vi "VannaSelection.vi"(2 "Vanna Motor":i16) -> (0 "Vanna Teleop Command":T1)   [LabVIEW 2019]
uses:
  Vanna Mode Type Def.ctl
  Vanna Command Type Def.ctl
panel:
  # "Operator Right joystick X: Vanna Manual. must have deadband.\nOperator Left Joystick Y: UP = Rotation control; DOWN = position control"
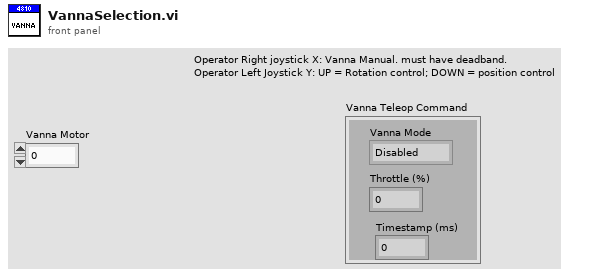
[diagram p1: front panel]
types:
  T1 = typedef "Vanna Command Type Def.ctl" = cluster{"Vanna Mode":T2, "Throttle (%)":dbl, "Timestamp (ms)":dbl}
  T2 = typedef "Vanna Mode Type Def.ctl" = enum16{"Disabled", "Raw Throttle", "Rotation Control", "Position Control"}
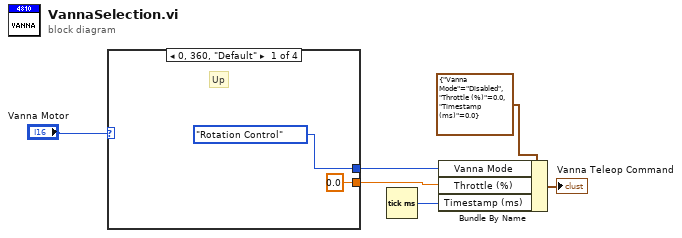
[diagram p0: block diagram]
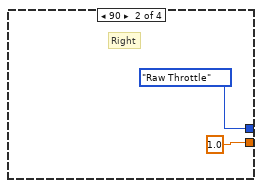
[diagram p2: hidden frame]
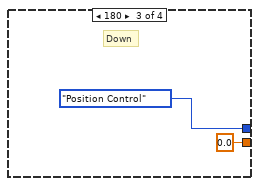
[diagram p3: hidden frame]
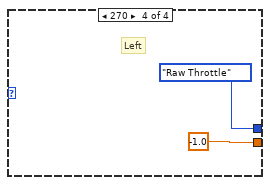
[diagram p4: hidden frame]
diagram:
  n1 = case shown="0, 360, \"Default\"" "Vanna Motor" {
    tunnel: [Vanna_Mode_Type_Def."Rotation Control" ("Vanna Mode") Vanna_Mode_Type_Def."Raw Throttle" ("Vanna Mode") Vanna_Mode_Type_Def."Position Control" ("Vanna Mode") Vanna_Mode_Type_Def."Raw Throttle" ("Vanna Mode")] -> w2
    tunnel: [0.0 ("Throttle (%)") 1.0 ("Throttle (%)") 0.0 ("Throttle (%)") -1.0 ("Throttle (%)")] -> w1
    frame 0, 360, 0 {
      # "Up"
    }
    frame 90 {
      # "Right"
    }
    frame 180 {
      # "Down"
    }
    frame 270 {
      # "Left"
    }
  }
  n2 = Tick Count (ms)() -> (millisecond timer value=w5:u32)
  n3 = Bundle By Name(cluster=T1 {"Vanna Mode"=enum."Disabled", "Throttle (%)"=0.0, "Timestamp (ms)"=0.0} ("Vanna Command"), "Vanna Mode"=w2, "Throttle (%)"=w1, "Timestamp (ms)"=w5) -> (→"Vanna Teleop Command":T1)
